vi "Communication - Initialize SV (SubVI).vi"(8 "error in (no error)":errorcluster) -> (0 "error out":errorcluster)   [LabVIEW 2019]
uses:
  Controls/Communication - Sensor Use.ctl
  Controls/Communication - LC PID.ctl
  Controls/Communication - TD PID.ctl
  Controls/FGV States.ctl
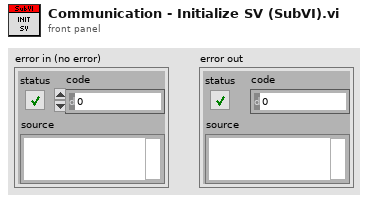
[diagram p1: front panel]
types:
  T1 = typedef "FGV States.ctl" = enum16{"Read", "Write"}
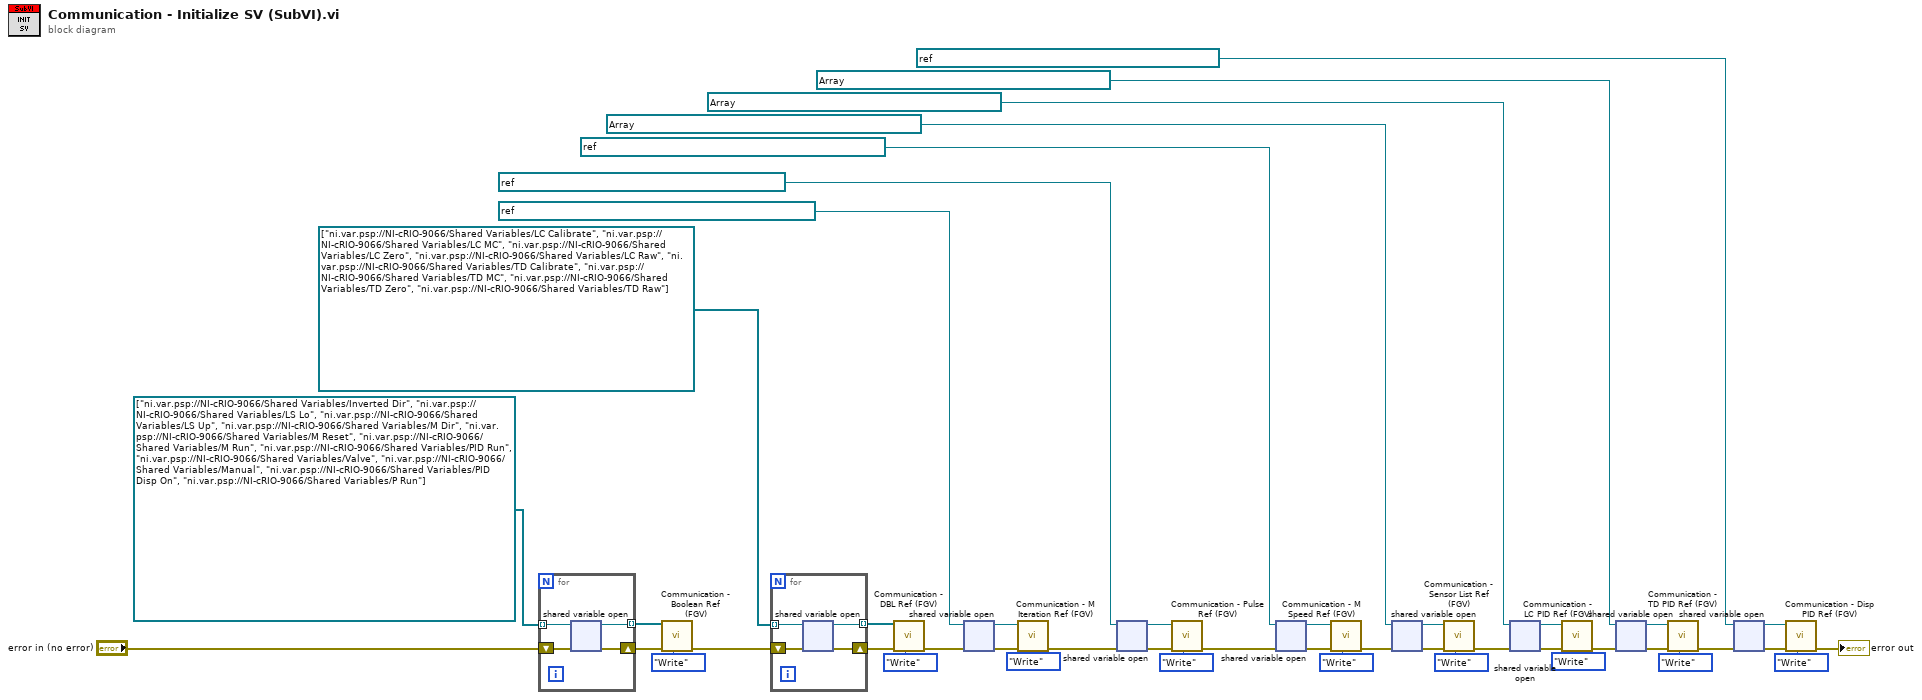
[diagram p0: block diagram]
diagram:
  w28 = refnum<k21> "ni.var.psp://NI-cRIO-9066/Shared Variables/Sensor List" items=["LC1", "LC2", "LC3", "LC4", "LC5", "LC6", "LC7", "LC8", "TD1", "TD2", "TD3", "TD4", "TD5", "TD6", "TD7", "TD8", "TD9", "TD10", "TD11", "TD12"] ("shared variable refnum in")
  n1 = for {
    tunnel: refnum<k21>[] ["ni.var.psp://NI-cRIO-9066/Shared Variables/Inverted Dir", "ni.var.psp://NI-cRIO-9066/Shared Variables/LS Lo", "ni.var.psp://NI-cRIO-9066/Shared Variables/LS Up", "ni.var.psp://NI-cRIO-9066/Shared Variables/M Dir", "ni.var.psp://NI-cRIO-9066/Shared Variables/M Reset", "ni.var.psp://NI-cRIO-9066/Shared Variables/M Run", "ni.var.psp://NI-cRIO-9066/Shared Variables/PID Run", "ni.var.psp://NI-cRIO-9066/Shared Variables/Valve", "ni.var.psp://NI-cRIO-9066/Shared Variables/Manual", "ni.var.psp://NI-cRIO-9066/Shared Variables/PID Disp On", "ni.var.psp://NI-cRIO-9066/Shared Variables/P Run"] -> [w48] mode=indexing
    shift-right: [w50] -> w44
    shift-left: "error in (no error)" -> [w49]
    tunnel: [w47] -> w45 mode=indexing
    n2 = shared-variable-open(w48, w49) -> (w47:refnum<k21>, w50:errorcluster)
  }
  n3 = call "Communication - Boolean Ref (FGV).vi"("Action"=FGV_States."Write", "error in (no error)"=w44, "Bool SV Ref"=w45) -> ("error out"=w39:errorcluster)  [unwired: 7 in, 1 out]
  n4 = for {
    tunnel: refnum<k21>[] ["ni.var.psp://NI-cRIO-9066/Shared Variables/LC Calibrate", "ni.var.psp://NI-cRIO-9066/Shared Variables/LC MC", "ni.var.psp://NI-cRIO-9066/Shared Variables/LC Zero", "ni.var.psp://NI-cRIO-9066/Shared Variables/LC Raw", "ni.var.psp://NI-cRIO-9066/Shared Variables/TD Calibrate", "ni.var.psp://NI-cRIO-9066/Shared Variables/TD MC", "ni.var.psp://NI-cRIO-9066/Shared Variables/TD Zero", "ni.var.psp://NI-cRIO-9066/Shared Variables/TD Raw"] -> [w52] mode=indexing
    shift-right: [w54] -> w41
    shift-left: w39 -> [w53]
    tunnel: [w51] -> w37 mode=indexing
    n5 = shared-variable-open(w52, w53) -> (w51:refnum<k21>, w54:errorcluster)
  }
  n6 = call "Communication - DBL Ref (FGV).vi"("Action"=FGV_States."Write", "error in (no error)"=w41, "SV DBL Ref"=w37) -> ("error out"=w36:errorcluster)  [unwired: 7 in, 1 out]
  n7 = shared-variable-open(refnum<k21> "ni.var.psp://NI-cRIO-9066/Shared Variables/M Iteration" ("shared variable refnum in"), w36) -> (w7:refnum<k21>, w35:errorcluster)
  n8 = call "Communication - M Iteration Ref (FGV).vi"("Action"=FGV_States."Write", "error in (no error)"=w35, "SV Iteration Ref"=w7) -> ("error out"=w6:errorcluster)  [unwired: 7 in, 1 out]
  n9 = shared-variable-open(refnum<k21> "ni.var.psp://NI-cRIO-9066/Shared Variables/Pulse" ("shared variable refnum in"), w6) -> (w3:refnum<k21>, w5:errorcluster)
  n10 = call "Communication - Pulse Ref (FGV).vi"("Action"=FGV_States."Write", "error in (no error)"=w5, "SV Iteration Ref"=w3) -> ("error out"=w4:errorcluster)  [unwired: 7 in, 1 out]
  n11 = shared-variable-open(refnum<k21> "ni.var.psp://NI-cRIO-9066/Shared Variables/M Speed" ("shared variable refnum in"), w4) -> (w30:refnum<k21>, w32:errorcluster)
  n12 = call "Communication - M Speed Ref (FGV).vi"("Action"=FGV_States."Write", "error in (no error)"=w32, "SV M Speed Ref"=w30) -> ("error out"=w29:errorcluster)  [unwired: 7 in, 1 out]
  n13 = shared-variable-open(w28, w29) -> (w27:refnum<k21>, w26:errorcluster)
  n14 = call "Communication - Sensor List Ref (FGV).vi"("Action"=FGV_States."Write", "error in (no error)"=w26, "SV Sensor List Ref"=w27) -> ("error out"=w24:errorcluster)  [unwired: 7 in, 1 out]
  n15 = shared-variable-open(refnum<k21> "ni.var.psp://NI-cRIO-9066/Shared Variables/LC PID" ("shared variable refnum in"), w24) -> (w19:refnum<k21>, w18:errorcluster)
  n16 = call "Communication - LC PID Ref (FGV).vi"("Action"=FGV_States."Write", "error in (no error)"=w18, "LC PID Ref"=w19) -> ("error out"=w17:errorcluster)  [unwired: 7 in, 1 out]
  n17 = shared-variable-open(refnum<k21> "ni.var.psp://NI-cRIO-9066/Shared Variables/TD PID" ("shared variable refnum in"), w17) -> (w15:refnum<k21>, w22:errorcluster)
  n18 = call "Communication - TD PID Ref (FGV).vi"("Action"=FGV_States."Write", "error in (no error)"=w22, "SV TD PID Ref"=w15) -> ("error out"=w14:errorcluster)  [unwired: 7 in, 1 out]
  n19 = shared-variable-open(refnum<k21> "ni.var.psp://NI-cRIO-9066/Shared Variables/Disp PID" ("shared variable refnum in"), w14) -> (w10:refnum<k21>, w12:errorcluster)
  n20 = call "Communication - Disp PID Ref (FGV).vi"("Action"=FGV_States."Write", "error in (no error)"=w12, "SV Disp PID Ref"=w10) -> ("error out"=→"error out":errorcluster)  [unwired: 7 in, 1 out]
